vi "Variant to Class.vi"(8 "error in (no error)":errorcluster, 10 "Data in":variant, 11 "Job Initialize in":refnum<class "Job Initialize.lvclass">) -> (0 "error out":errorcluster, 2 "Data Out":variant, 3 "Job Initialize out":refnum<class "Job Initialize.lvclass">)   [LabVIEW 2014, in "Job Initialize.lvclass"]
uses:
  Job Initialize.lvclass
  Job Initialize.lvclass/Job Initialize.ctl
  Build Job/Build Job.lvclass
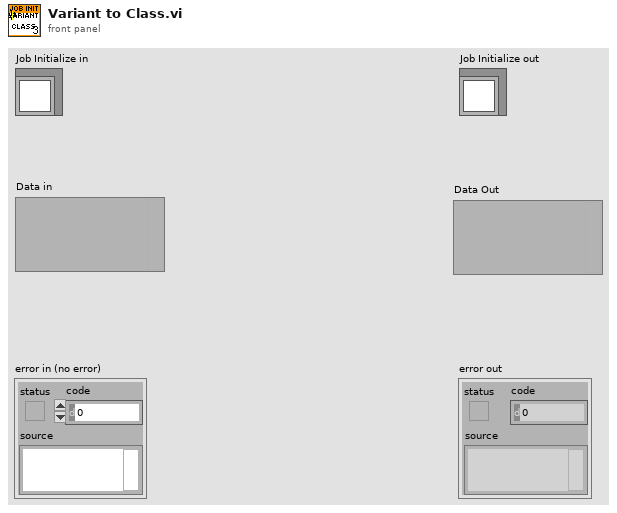
[diagram p1: front panel]
types:
  T1 = typedef "Cron String - STYP.ctl" = cluster{"Day of Week":enum16{"Everyday", "Sunday", "Monday", "Tuesday", "Wednesday", "Thursday", "Friday", "Saturday"}, "Hour":i32, "Enable?":bool}
  T2 = typedef "Source Code Control Selection - STYP.ctl" = enum16{"None (Manual Build)", "Every 15 Minutes", "Every 30 Minutes", "Every 45 Minutes", "Every Hour", "Every 2 Hours", "Everyday "}
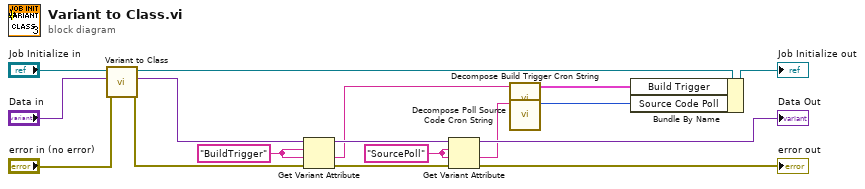
[diagram p0: block diagram]
diagram:
  w9 = "SourcePoll" ("name")
  w11 = "BuildTrigger" ("name")
  n1 = call-parent "Variant to Class.vi"("error in (no error)"="error in (no error)", "Data in"="Data in", "Build Job in"="Job Initialize in") -> ("error out"=w8:errorcluster, "Data Out"=w12:variant, "Build Job out"=w14:refnum<class "Job Initialize.lvclass">)  [unwired: 6 in]
  n2 = Get Variant Attribute(Variant=w12, name=w11, default value (empty Variant)=w11, error in=w8) -> (duplicate Variant=w10:variant, value=w1:string, error out=w7:errorcluster)  [unwired: 1 out]
  n3 = Get Variant Attribute(Variant=w10, name=w9, default value (empty Variant)=w9, error in=w7) -> (duplicate Variant=→"Data Out":variant, value=w4:string, error out=→"error out":errorcluster)  [unwired: 1 out]
  n4 = call "Decompose Build Trigger Cron String.vi"("String"=w1) -> ("Cron Cluster"=w2:T1)  [unwired: 10 in]
  n5 = call "Decompose Poll Source Code Cron String.vi"("String"=w4) -> ("Source Code Poll"=w3:T2)  [unwired: 10 in]
  n6 = Bundle By Name(cluster=w14, "Build Trigger"=w2, "Source Code Poll"=w3) -> (→"Job Initialize out":refnum<class "Job Initialize.lvclass">)
